vi "Get Game Board.vi"(8 "error in (no error)":errorcluster caption="entrée d'erreur (pas d'erreur)", 11 "Game Board en entrée":refnum<class "Game Board.lvclass">) -> (0 "error out":errorcluster caption="sortie d'erreur", 2 "Game Board":u32[][](array[numeric]), 3 "Game Board en sortie":refnum<class "Game Board.lvclass">)   [LabVIEW 2017, in "Game Board.lvclass"]
uses:
  Game Board.lvclass
  Game Board.lvclass/Game Board.ctl
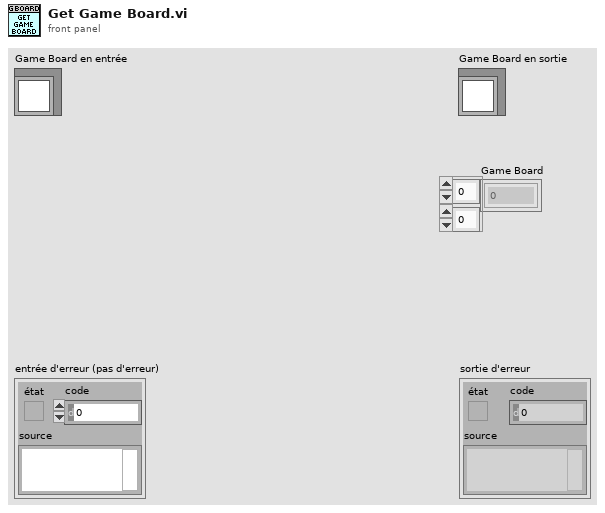
[diagram p1: front panel]
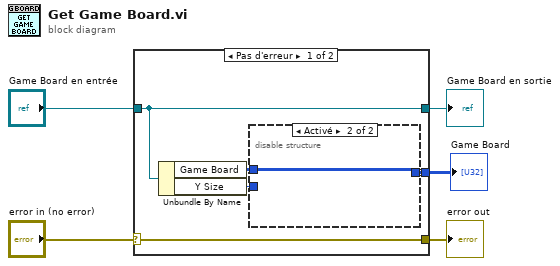
[diagram p0: block diagram]
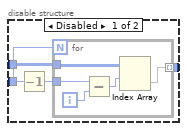
[diagram p2: hidden frame]
diagram:
  n1 = case shown="Pas d'erreur" "error in (no error)" {
    selector: "error in (no error)" -> [w10 w22]
    tunnel: [w10 w22] -> w4
    tunnel: [w9 w21] -> w2
    tunnel: "Game Board en entrée" -> [w9 w21]
    tunnel: [w6 _] -> w1
    frame No Error {
      n2 = Unbundle By Name(w9) -> ("Game Board"=w8:u32[][], "Y Size"=w7:i32)
      n3 = disable-structure shown="Activé" {
        disable-tunnel: w8 -> [w14 w20]
        disable-tunnel: w7 -> [w13 _]
        disable-tunnel: [w12 w20] -> w6
        frame Disabled {
          n4 = Decrement(x=w13) -> (x-1=w11:i32)
          n5 = for {
            N: w13 -> [_]
            tunnel: w14 -> [w19]
            tunnel: w11 -> [w18]
            tunnel: [w15] -> w12 mode=indexing
            i -> [w17]
            n6 = Subtract(x=w18, y=w17) -> (x-y=w16:i32)
            n7 = Index Array(array=w19, index (row)=w16) -> (element=w15:u32[])  [unwired: 1 in]
          }
        }
        frame Enabled {
        }
      }
    }
    frame Error {
    }
  }
  "error out" <- w4
  "Game Board en sortie" <- w2
  "Game Board" <- w1
